vi "get polarization.vi"() -> ()   [LabVIEW 2018]
panel:
  in  "max":dbl
  in  "min":dbl
  in  "background intensity":dbl
  out "estimated polarization":dbl
  in  "polarimeter angle":dbl
  in  "pressure factor":dbl
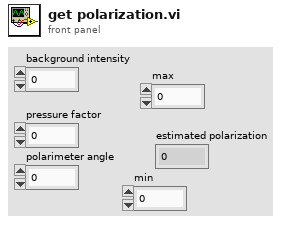
[diagram p1: front panel]
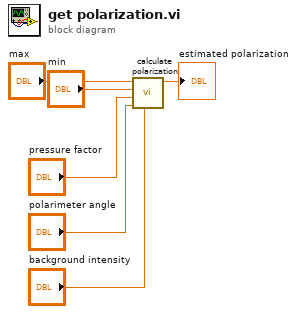
[diagram p0: block diagram]
diagram:
  n1 = call "calculate polarization.vi"("background intensity"="background intensity", "polarimeter angle"="polarimeter angle", "pressure factor"="pressure factor", "min"="min", "max"="max") -> ("estimated polarization"=→"estimated polarization":dbl)  [unwired: 6 in]
